vi "_toString.vi"(8 "error in (no error)":errorcluster, 11 "Record.Error in":refnum<class "Record.Error.lvclass">) -> (0 "error out":errorcluster, 2 "String":string, 3 "Record.Error out":refnum<class "Record.Error.lvclass">)   [LabVIEW 2017, in "Error Log.lvlib" / "Record.Error.lvclass"]
uses:
  Record.Error.lvclass
  <vilib>/addons/_JKI.lib/Serialization/JSON/JKI JSON Serialization.lvlib
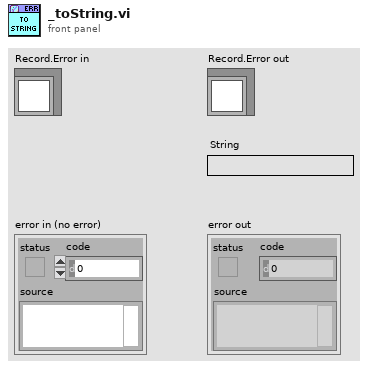
[diagram p1: front panel]
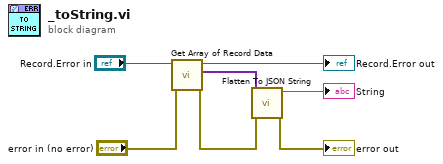
[diagram p0: block diagram]
diagram:
  n1 = call-dynamic "Get Array of Record Data.vi"("error in (no error)"="error in (no error)", "Record.Error in"="Record.Error in") -> ("error out"=w3:errorcluster, "Array of Record Data"=w4:variant[], "Record.Error out"=→"Record.Error out":refnum<class "Record.Error.lvclass">)  [unwired: 7 in]
  n2 = call <vilib>:"Flatten To JSON String.vi"("error in (no error)"=w3, "Variant"=w4) -> ("error out"=→"error out":errorcluster, "JSON String"=→"String":string)  [unwired: 8 in]
